vi "Send Single Pusle.vi"(8 "error in (no error)":errorcluster, 10 "Action Data":variant, 11 "Controller in":refnum<class "Controller.lvclass">) -> (0 "error out":errorcluster)   [LabVIEW 2020, in "Controller.lvlib" / "Controller.lvclass"]
uses:
  Controller.lvclass
  Actor_Scope/Actor_Scope/Scope_Action.ctl
  Controller.lvclass/Controller.ctl
  Actor_AFG/Actor_AFG Messages/Setup Pulse Waveform Msg/Setup Pulse Waveform Msg.lvclass/Setup Pulse Waveform Msg.ctl
  <vilib>/ActorFramework/Message Enqueuer/Message Enqueuer.lvclass/Message Enqueuer.ctl
  Actor_AFG/Actor_AFG Messages/AFG Setup Cycle Msg/AFG Setup Cycle Msg.lvclass/AFG Setup Cycle Msg.ctl
  Actor_AFG/Actor_AFG Messages/AFG Enable Output Msg/AFG Enable Output Msg.lvclass/AFG Enable Output Msg.ctl
  Actor_Scope/Actor_Scope Messages/Do Scope Action Msg/Do Scope Action Msg.lvclass/Do Scope Action Msg.ctl
  <vilib>/ActorFramework/Message Enqueuer/Enqueue.vi
  Actor_AFG/Actor_AFG Messages/Setup Pulse Waveform Msg/Setup Pulse Waveform Msg.lvclass
  C:/Program Files/National Instruments/LabVIEW 2020/vi.lib/ActorFramework/Message/Message.lvclass
  Actor_AFG/Actor_AFG Messages/AFG Setup Cycle Msg/AFG Setup Cycle Msg.lvclass
  Actor_AFG/Actor_AFG Messages/AFG Enable Output Msg/AFG Enable Output Msg.lvclass
  Actor_Scope/Actor_Scope Messages/Do Scope Action Msg/Do Scope Action Msg.lvclass
  Actor_NI6008/Actor_NI6008 Messages/NI6008 Enout Trigger Msg/NI6008 Enout Trigger Msg.lvclass
  <vilib>/ActorFramework/Message Priority Queue/Priority Enqueue.vi
  Actor_Scope/Actor_Scope/Actor_Scope.lvclass
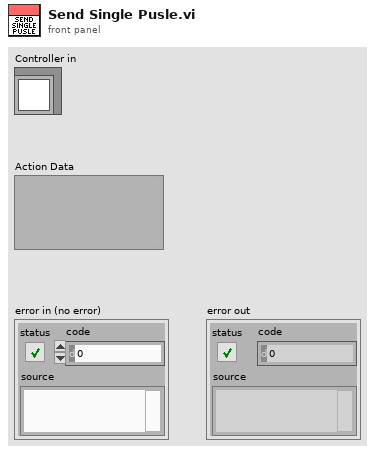
[diagram p1: front panel]
types:
  T1 = typedef "Actor_Scope.lvlib/Actor_Scope.lvclass/Scope_Action.ctl" = enum16{"Config Trigger", "Init Wfm Acq", "Read Wfm"}
  T2 = cluster{"Set Pulse Conf":cluster{"V Conf":cluster{"Bias":dbl, "Amp":dbl}, "T Conf":cluster{"Rise Time":dbl, "Fall Time":dbl, "Pulse Width":dbl}}, "Reset Pulse Conf":cluster{"V Conf":cluster{"Bias":dbl, "Amp":dbl}, "T Conf":cluster{"Rise Time":dbl, "Fall Time":dbl, "Pulse Width":dbl}}}
  T3 = cluster{"V Conf":cluster{"Bias":dbl, "Amp":dbl}, "T Conf":cluster{"Rise Time":dbl, "Fall Time":dbl, "Pulse Width":dbl}}
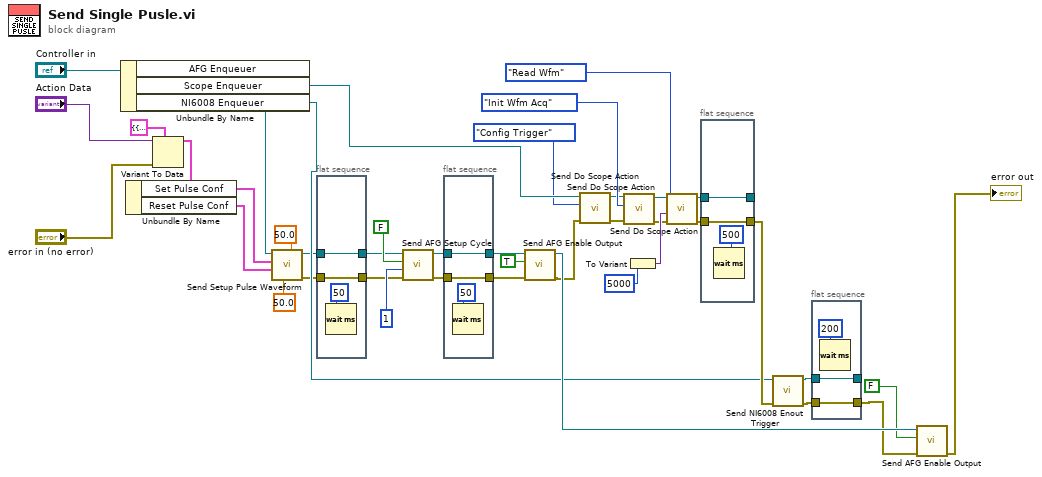
[diagram p0: block diagram]
diagram:
  n1 = Unbundle By Name("Controller in") -> ("AFG Enqueuer"=w16:refnum<class "Message Enqueuer.lvclass">, "Scope Enqueuer"=w30:refnum<class "Message Enqueuer.lvclass">, "NI6008 Enqueuer"=w35:refnum<class "Message Enqueuer.lvclass">)
  n2 = Variant To Data(error in="error in (no error)", type=T2 {"Set Pulse Conf"={"V Conf"={"Bias"=1.0, "Amp"=2.5}, "T Conf"={"Rise Time"=5.0, "Fall Time"=5.0, "Pulse Width"=20.0}}, "Reset Pulse Conf"={"V Conf"={"Bias"=-0.5, "Amp"=-2.5}, "T Conf"={"Rise Time"=5.0, "Fall Time"=5.0, "Pulse Width"=20.0}}}, Variant="Action Data") -> (data=w12:T2)  [unwired: 1 out]
  n3 = Unbundle By Name(w12) -> ("Set Pulse Conf"=w13:T3, "Reset Pulse Conf"=w14:T3)
  n4 = call "Send Setup Pulse Waveform.vi"("Spacing"=50.0, "Delay"=50.0, "Reset Pulse Conf"=w14, "Set Pulse Conf"=w13, "Message Enqueuer"=w16) -> ("error out"=w9:errorcluster, "Message Enqueuer out"=w6:refnum<class "Message Enqueuer.lvclass">)  [unwired: 5 in]
  n5 = flat-sequence {
    tunnel: w6 -> [w45]
    tunnel: [w45] -> w7
    tunnel: [w44] -> w8
    tunnel: w9 -> [w44]
    frame #0 {
      n6 = Wait (ms)(milliseconds to wait=u32 50) -> ()  [unwired: 1 out]
    }
  }
  n7 = call "Send AFG Setup Cycle.vi"("error in (no error)"=w8, "Cycles"=1 ("Cycle"), "Continuous"=FALSE ("Repeat"), "Message Enqueuer"=w7) -> ("error out"=w18:errorcluster, "Message Enqueuer out"=w17:refnum<class "Message Enqueuer.lvclass">)  [unwired: 6 in]
  n8 = flat-sequence {
    tunnel: w17 -> [w47]
    tunnel: w18 -> [w46]
    tunnel: [w47] -> w19
    tunnel: [w46] -> w32
    frame #0 {
      n9 = Wait (ms)(milliseconds to wait=u32 50) -> ()  [unwired: 1 out]
    }
  }
  n10 = call "Send AFG Enable Output.vi"("error in (no error)"=w32, "Enable Output (T: Enable)"=TRUE, "Message Enqueuer"=w19) -> ("error out"=w31:errorcluster, "Message Enqueuer out"=w41:refnum<class "Message Enqueuer.lvclass">)  [unwired: 7 in]
  n11 = call "Send Do Scope Action.vi"("error in (no error)"=w31, "Scope Action"=Scope_Action."Config Trigger", "Message Enqueuer"=w30) -> ("error out"=w23:errorcluster, "Message Enqueuer out"=w22:refnum<class "Message Enqueuer.lvclass">)  [unwired: 7 in]
  n12 = call "Send Do Scope Action.vi"("error in (no error)"=w23, "Scope Action"=Scope_Action."Init Wfm Acq", "Message Enqueuer"=w22) -> ("error out"=w26:errorcluster, "Message Enqueuer out"=w25:refnum<class "Message Enqueuer.lvclass">)  [unwired: 7 in]
  n13 = To Variant(anything=5000 ("Time Out (ms)")) -> (Variant=w29:variant)
  n14 = call "Send Do Scope Action.vi"("error in (no error)"=w26, "Action Data In"=w29, "Scope Action"=Scope_Action."Read Wfm", "Message Enqueuer"=w25) -> ("error out"=w34:errorcluster, "Message Enqueuer out"=w33:refnum<class "Message Enqueuer.lvclass">)  [unwired: 6 in]
  n15 = flat-sequence {
    tunnel: w33 -> [w50]
    tunnel: w34 -> [w49]
    tunnel: [w50] -> _
    tunnel: [w49] -> w36
    frame #0 {
      n16 = Wait (ms)(milliseconds to wait=u32 500) -> ()  [unwired: 1 out]
    }
  }
  n17 = call "Send NI6008 Enout Trigger.vi"("error in (no error)"=w36, "Message Enqueuer"=w35) -> ("error out"=w38:errorcluster, "Message Enqueuer out"=w37:refnum<class "Message Enqueuer.lvclass">)  [unwired: 8 in]
  n18 = flat-sequence {
    tunnel: w37 -> [w53]
    tunnel: w38 -> [w52]
    tunnel: [w53] -> _
    tunnel: [w52] -> w39
    frame #0 {
      n19 = Wait (ms)(milliseconds to wait=u32 200) -> ()  [unwired: 1 out]
    }
  }
  n20 = call "Send AFG Enable Output.vi"("error in (no error)"=w39, "Enable Output (T: Enable)"=FALSE, "Message Enqueuer"=w41) -> ("error out"=→"error out":errorcluster)  [unwired: 7 in, 1 out]
